vi "Remove Value.vi"(8 "error in (no error)":errorcluster, 10 "key":string, 11 "JSON Value in":refnum<class "JSON Value.lvclass">) -> (0 "error out":errorcluster, 2 "found":bool, 3 "JSON Value out":refnum<class "JSON Value.lvclass">)   [LabVIEW 2016, in "JSON Value.lvclass"]
doc: "Remove the given parameter from the specified JSON Object"
uses:
  JSON Value.lvclass
  JSON Value.lvclass/JSON Value.ctl
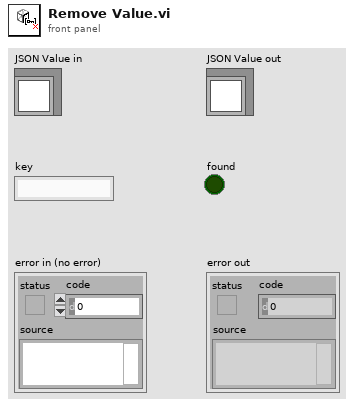
[diagram p1: front panel]
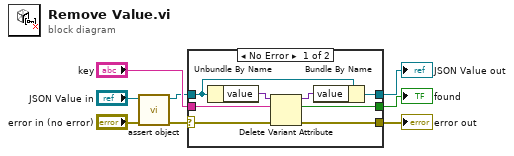
[diagram p0: block diagram]
diagram:
  n1 = call "assert object.vi"("error in (no error)"="error in (no error)", "JSON Value in"="JSON Value in") -> ("error out"=w3:errorcluster, "JSON Value out"=w1:refnum<class "JSON Value.lvclass">)  [unwired: 8 in]
  n2 = case shown="No Error" w3 {
    selector: w3 -> [w15 w18]
    tunnel: [w13 w18] -> w7
    tunnel: w1 -> [w11 w17]
    tunnel: "key" -> [w16 _]
    tunnel: [w12 _] -> w5
    tunnel: [w9 w17] -> w4
    frame No Error {
      n3 = Unbundle By Name(w11) -> ("value"=w14:variant)
      n4 = Delete Variant Attribute(4:w15, 6:w16, 7:w14) -> (0:w13:errorcluster, 2:w12:bool, 3:w10:variant)
      n5 = Bundle By Name(cluster=w11, "value"=w10) -> (w9:refnum<class "JSON Value.lvclass">)
    }
    frame Error {
    }
  }
  "error out" <- w7
  "found" <- w5
  "JSON Value out" <- w4
